vi "Main.vi"() -> ()   [LabVIEW 2012]
doc: "This sample project is built upon the standard state machine template and shows how you could create an application that acquires, analyzes, and presents data. It includes functionality for presenting configuration dialogs, preserving settings between executions, loading and saving data, as well as exporting graph images and text files.\n\nIt is most appropriate for data that is acquired instantly as it does not allow for screen updates mid acquisition nor does it allow for continuous streaming to disk."
uses:
  controls/State.ctl
  controls/Data.ctl
  controls/UI References.ctl
  controls/Graph Data.ctl
  <vilib>/Utility/miscctls.llb/LVAnnotationListTypeDef.ctl
  <vilib>/Utility/miscctls.llb/LVCursorListTypeDef.ctl
  controls/User Specified Data.ctl
  controls/HW Configuration.ctl
  controls/Simulated Signal Type.ctl
  controls/Analysis Configuration.ctl
  controls/New Data Behavior.ctl
  <resource>/Framework/Providers/Wirebird Labs LLC/Deploy/Support/Release Class/Deploy-UpdateService-PromptLevel.ctl
  <resource>/Framework/Providers/Wirebird Labs LLC/Deploy/Support/Update Watcher Class/Deploy-UpdateWatcher.lvclass
  <resource>/Framework/Providers/Wirebird Labs LLC/Deploy/Support/Release Class/Deploy-Release.lvclass
panel:
  in  "Settings":bool
  in  "Snapshot":bool
  in  "Analyze":bool
  in  "Clear":bool
  in  "Stop":bool
  in  "Acquire":bool
  in  "Export":bool
  in  "Save Data":bool
  in  "Load Data":bool
  out "Graph":waveform(dbl)[](graph)
  out "Status Bar":string
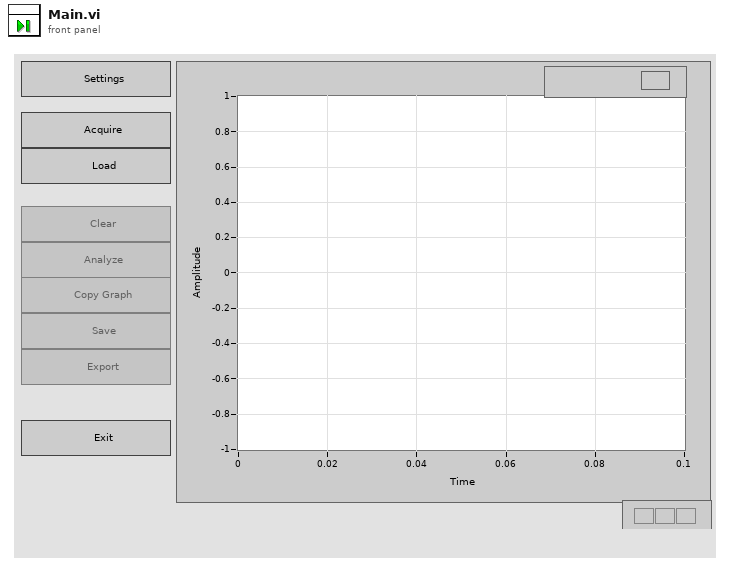
[diagram p1: front panel]
types:
  T1 = typedef "Deploy-Release.lvclass/Deploy-UpdateService-PromptLevel.ctl" = enum16{"Prompt User", "Auto (Show Progress Only)"}
  T2 = typedef "Data.ctl" = cluster{"UI References":T3, "Graph Data":T4, "User Specified":T7}
  T3 = typedef "UI References.ctl" = cluster{"Stop Ref":refnum<vi>, "Save Ref":refnum<vi>, "Open Ref":refnum<vi>, "Export Ref":refnum<vi>, "Acquire Ref":refnum<vi>, "Configure Ref":refnum<vi>, "Graph Ref":refnum<vi>, "Clear Ref":refnum<vi>, "Analyze Ref":refnum<vi>, "Status Ref":refnum<vi>, "Snapshot Ref":refnum<vi>}
  T4 = typedef "Graph Data.ctl" = cluster{"Data":waveform(dbl)[], "Annotation List":T5, "Cursor List":T6, "Analysis Data":waveform(dbl)[]}
  T5 = typedef "LVAnnotationListTypeDef.ctl" = cluster{"Name":string, "Color":u32, "Style":u8, "Point Style":u8, "Name Visible":bool, "Allow Drag":bool, "Annotation Mode":u32, "Plot":i32, "Index":i32, "Position":cluster{"X":dbl, "Y":dbl}, "X Scale":u32, "Y Scale":u32, "Show Arrow":bool, "Lock Name":bool, "Plot Area":i32, "Label Offset":cluster{"X":dbl, "Y":dbl}}[]
  T6 = typedef "LVCursorListTypeDef.ctl" = cluster{"Name":string, "Color":u32, "Style":u8, "Point Style":u8, "Name Visible":bool, "Allow Drag":bool, "Cursor Mode":u32, "Plot":i32, "Index":i32, "Position":cluster{"X":dbl, "Y":dbl}, "X Scale":u32, "Y Scale":u32, "Watch Plots":i32[], "Watch All Plots":bool, "Plot Area":i32, "Label Offset":cluster{"X":dbl, "Y":dbl}}[]
  T7 = typedef "User Specified Data.ctl" = cluster{"Hardware Configuration":T8, "Analysis Configuration":T10, "New Data Behavior":T11}
  T8 = typedef "HW Configuration.ctl" = cluster{"HW Refnum <Replace Me>":string, "Signal Type <Replace Me>":T9}
  T9 = typedef "Simulated Signal Type.ctl" = enum16{"Sine Wave", "Square Wave"}
  T10 = typedef "Analysis Configuration.ctl" = cluster{"Statistics":bool}
  T11 = typedef "New Data Behavior.ctl" = enum16{"Replace", "Overlay", "Append"}
  T12 = typedef "State.ctl" = enum16{"Initialize", "Wait for Event", "Update UI", "Configure", "Acquire", "Load Data", "Save Data", "Clear Data", "Export Data", "Analyze", "Copy Graph", "Stop"}
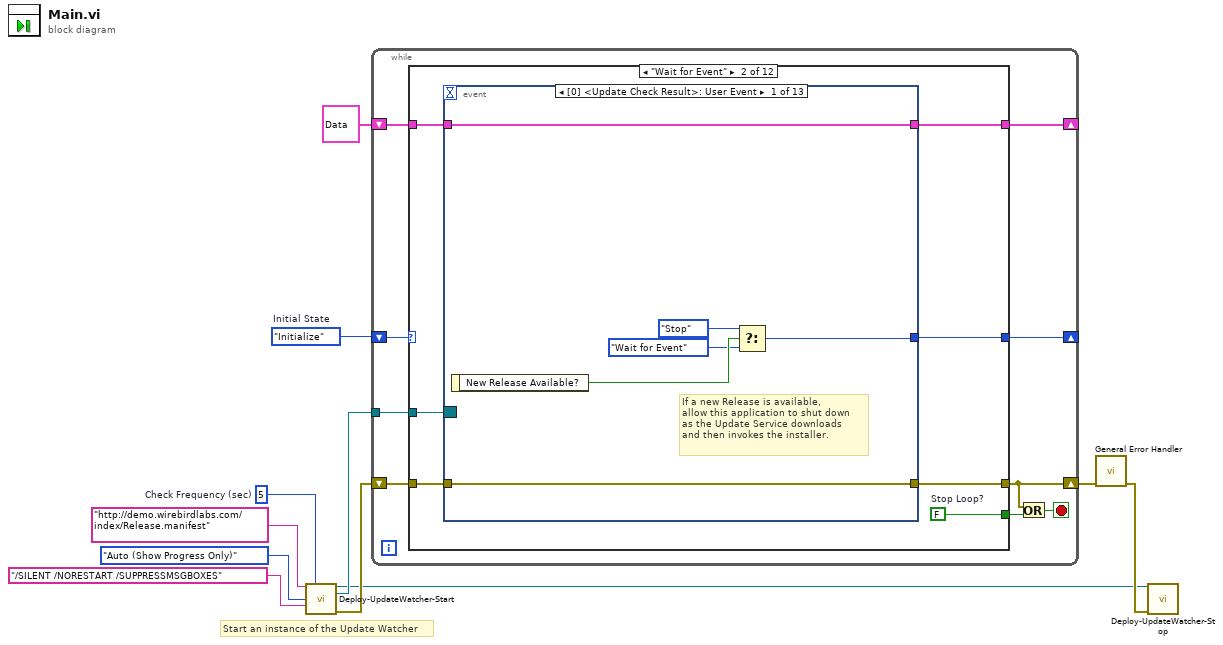
[diagram p0: block diagram]
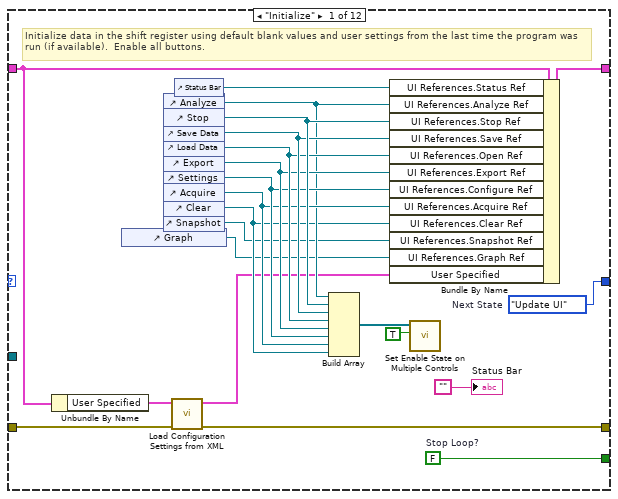
[diagram p2: hidden frame]
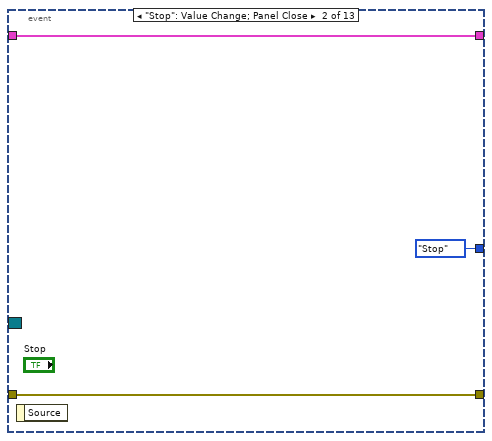
[diagram p3: hidden frame]
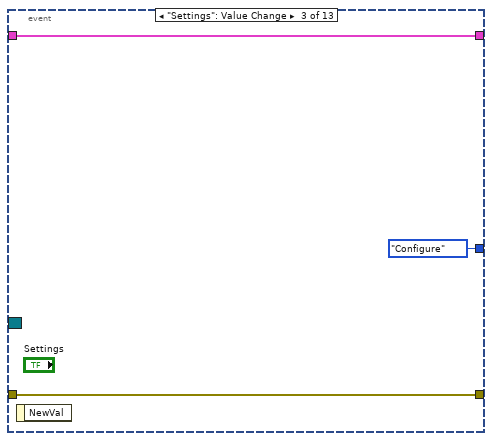
[diagram p4: hidden frame]
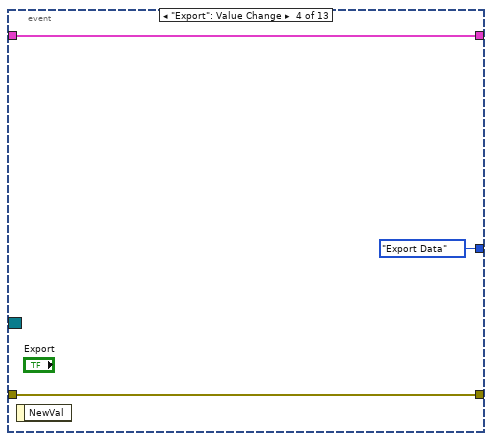
[diagram p5: hidden frame]
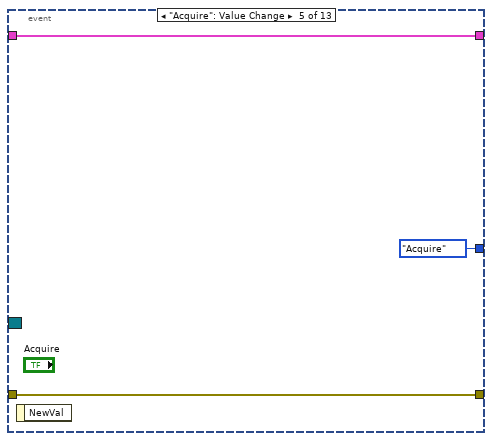
[diagram p6: hidden frame]
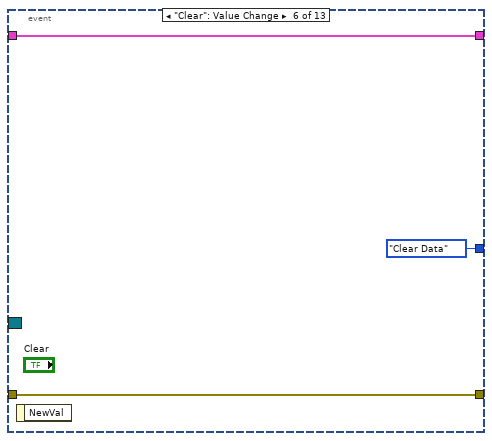
[diagram p7: hidden frame]
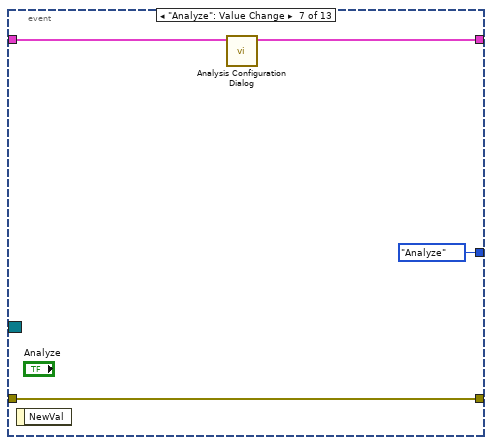
[diagram p8: hidden frame]
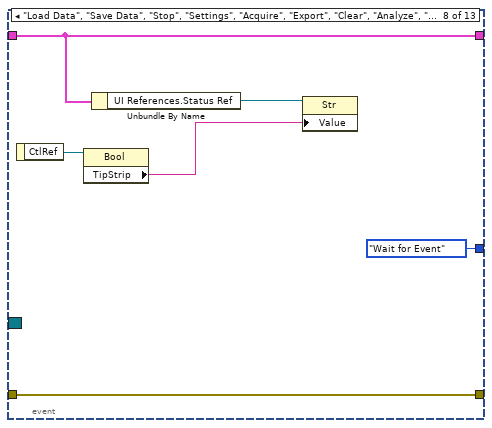
[diagram p9: hidden frame]
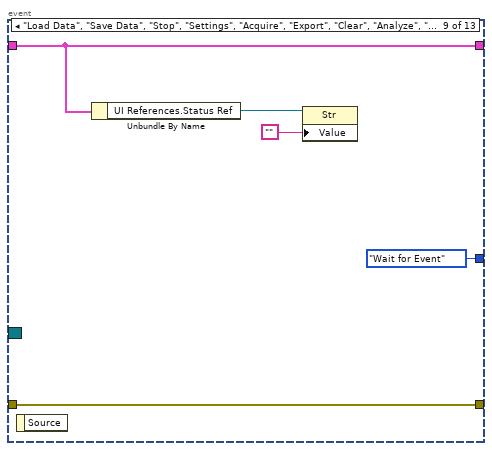
[diagram p10: hidden frame]
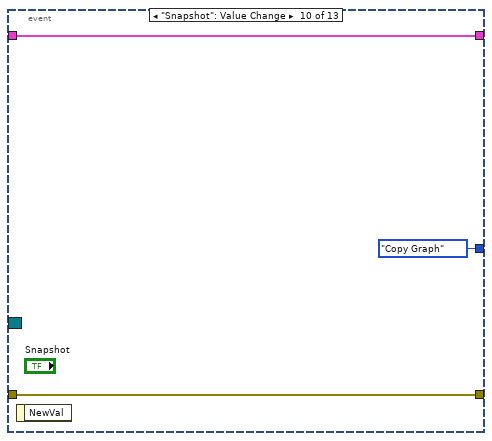
[diagram p11: hidden frame]
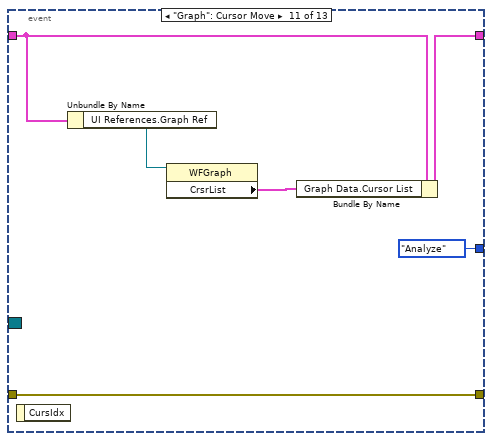
[diagram p12: hidden frame]
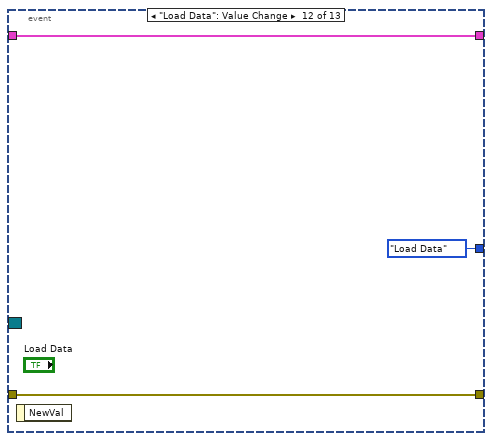
[diagram p13: hidden frame]
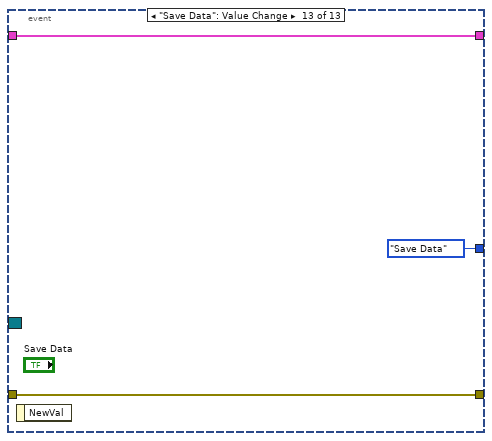
[diagram p14: hidden frame]
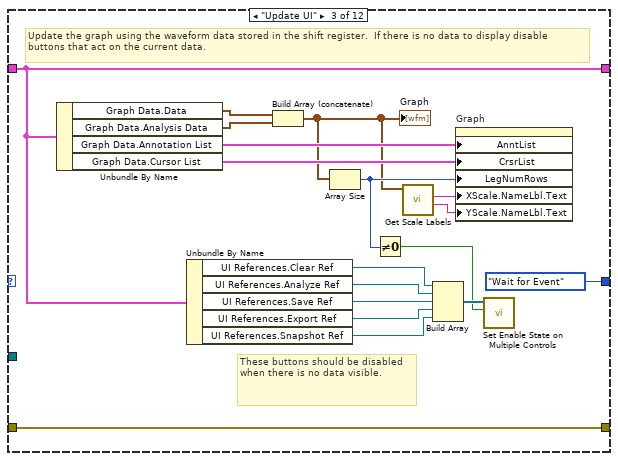
[diagram p15: hidden frame]
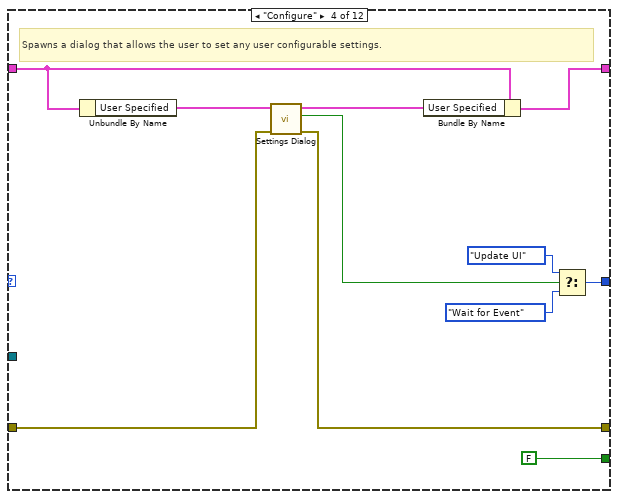
[diagram p16: hidden frame]
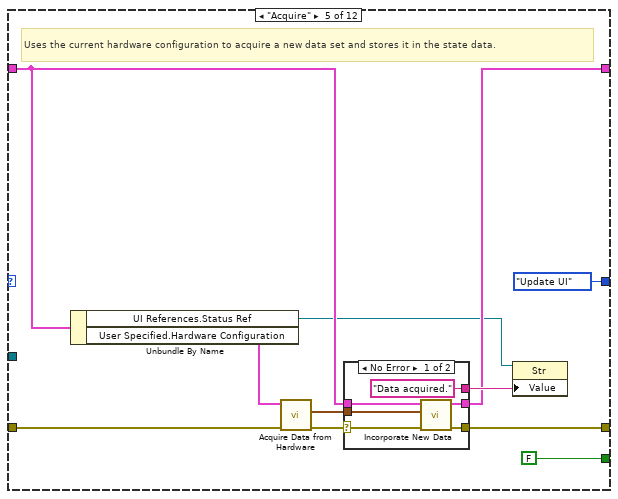
[diagram p17: hidden frame]
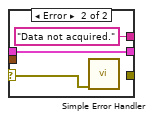
[diagram p18: hidden frame]
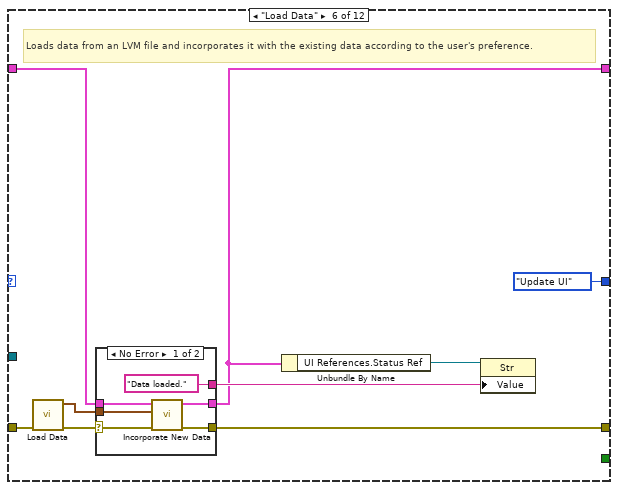
[diagram p19: hidden frame]
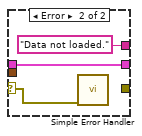
[diagram p20: hidden frame]
diagram:
  w2 = 5  # Check Frequency (sec)
  w11 = State."Initialize"  # Initial State
  # "Start an instance of the Update Watcher"
  n1 = call <resource>:"Deploy-UpdateWatcher-Start.vi"("Manifest URI"="http://demo.wirebirdlabs.com/index/Release.manifest", "Check Frequency (sec)"=w2, "Prompt Level"=Deploy-UpdateService-PromptLevel."Auto (Show Progress Only)", "Installer Command Line Parameters"="/SILENT /NORESTART /SUPPRESSMSGBOXES") -> (4:"Update Watcher"=w3:refnum<class "Deploy-UpdateWatcher.lvclass">, 6:"Update Watcher"=w8:refnum<event-registration>, "error out"=w6:errorcluster)  [unwired: 9 in]
  n2 = while {
    shift-right: [w19] -> _
    shift-left: w11 -> [w20]
    shift-right: [w17] -> _
    shift-left: T2 {"UI References"={"Stop Ref"=refnum, "Save Ref"=refnum, "Open Ref"=refnum, "Export Ref"=refnum, "Acquire Ref"=refnum, "Configure Ref"=refnum, "Graph Ref"=refnum, "Clear Ref"=refnum, "Analyze Ref"=refnum, "Status Ref"=refnum, "Snapshot Ref"=refnum}, "Graph Data"={"Data"=[], "Annotation List"=[], "Cursor List"=[], "Analysis Data"=[]}, "User Specified"={"Hardware Configuration"={"HW Refnum <Replace Me>"="", "Signal Type <Replace Me>"=enum."Sine Wave"}, "Analysis Configuration"={"Statistics"=FALSE}, "New Data Behavior"=enum."Replace"}} ("Data") -> [w18]
    shift-right: [w13] -> w9
    shift-left: w6 -> [w16]
    tunnel: w8 -> [w12]
    stop <- w14 stop-if-true
    n3 = case shown="\"Wait for Event\"" w20 {
      tunnel: [w42 w49 State."Wait for Event" ("(Value Not Used)") w122 State."Update UI" ("Next State") State."Update UI" ("(Value Not Used)") State."Wait for Event" ("(Value Not Used)") State."Wait for Event" ("(Value Not Used)") State."Update UI" ("(Value Not Used)") State."Update UI" ("(Value Not Used)") State."Wait for Event" ("(Value Not Used)") w212] -> w19
      tunnel: [w41 w48 _ FALSE ("Stop Loop?") FALSE ("Stop Loop?") _ _ _ _ _ _ w211] -> w15
      tunnel: w18 -> [w32 w47 w115 w128 w135 w158 w171 w183 w194 w197 w203 w209]
      tunnel: [w40 w46 w115 w127 w134 w152 w171 w183 w193 w197 w203 w209] -> w17
      tunnel: w16 -> [w30 w45 w118 w126 w137 w157 w173 w186 w196 w198 w202 w206]
      tunnel: [w29 w44 w118 w125 w130 w156 w169 w180 w196 w198 w201 w205] -> w13
      tunnel: w12 -> [_ w43 _ _ _ _ _ _ _ _ _ _]
      frame "Initialize" {
        w41 = FALSE  # Stop Loop?
        w42 = State."Update UI"  # Next State
        # "Initialize data in the shift register using default blank values and user settings from the last time the program was run (if available).  Enable all buttons."
        n4 = Unbundle By Name(w32) -> ("User Specified"=w31:T7)
        n5 = control-ref of="Graph"() -> (w21:refnum<vi>)
        n6 = control-ref of="Analyze"() -> (w28:refnum<vi>)
        n7 = control-ref of="Stop"() -> (w39:refnum<vi>)
        n8 = control-ref of="Save Data"() -> (w38:refnum<vi>)
        n9 = control-ref of="Load Data"() -> (w37:refnum<vi>)
        n10 = control-ref of="Export"() -> (w36:refnum<vi>)
        n11 = control-ref of="Settings"() -> (w35:refnum<vi>)
        n12 = control-ref of="Acquire"() -> (w34:refnum<vi>)
        n13 = control-ref of="Clear"() -> (w26:refnum<vi>)
        n14 = control-ref of="Snapshot"() -> (w22:refnum<vi>)
        n15 = call "Load Configuration Settings from XML.vi"("error in (no error)"=w30, "User Configuration in"=w31) -> ("error out"=w29:errorcluster, "User Configuration out"=w24:T7)  [unwired: 8 in]
        n16 = control-ref of="Status Bar"() -> (w27:refnum<vi>)
        n17 = Build Array(w28, w39, w38, w37, w36, w35, w34, w26) -> (w33:refnum<vi>[])
        n18 = Bundle By Name(cluster=w32, "UI References.Status Ref"=w27, "UI References.Analyze Ref"=w28, "UI References.Stop Ref"=w39, "UI References.Save Ref"=w38, "UI References.Open Ref"=w37, "UI References.Export Ref"=w36, "UI References.Configure Ref"=w35, "UI References.Acquire Ref"=w34, "UI References.Clear Ref"=w26, "UI References.Snapshot Ref"=w22, "UI References.Graph Ref"=w21, "User Specified"=w24) -> (w40:T2)
        n19 = call "Set Enable State on Multiple Controls.vi"("Enable?"=TRUE, "Controls"=w33) -> ()  [unwired: 10 in]
        "Status Bar" <- "" ("Status Bar")
      }
      frame "Wait for Event" {
        w48 = FALSE  # Stop Loop?
        n20 = event shown="[0] <Update Check Result>: User Event" {
          selector: w43 -> [_ _ _ _ _ _ _ _ _ _ _ _ _]
          dyn-events: _ -> [_ _ _ _ _ _ _ _ _ _ _ _ _]
          timeout: _ -> [_ _ _ _ _ _ _ _ _ _ _ _ _]
          tunnel: [w51 State."Stop" ("Next State") State."Configure" ("Next State") State."Export Data" ("Next State") State."Acquire" ("Next State") State."Clear Data" ("Next State") State."Analyze" ("Next State") State."Wait for Event" ("Next State") State."Wait for Event" ("Next State") State."Copy Graph" ("Next State") State."Analyze" ("Next State") State."Load Data" ("Next State") State."Save Data" ("Next State")] -> w49
          tunnel: w47 -> [w55 w57 w61 w64 w67 w70 w72 w78 w84 w88 w89 w96 w99]
          tunnel: [w55 w57 w61 w64 w67 w70 w71 w78 w84 w88 w92 w96 w99] -> w46
          tunnel: w45 -> [w54 w56 w60 w63 w66 w69 w74 w80 w85 w87 w94 w95 w98]
          tunnel: [w54 w56 w60 w63 w66 w69 w74 w80 w85 w87 w94 w95 w98] -> w44
          event User Event {
            # "If a new Release is available,\nallow this application to shut down\nas the Update Service downloads\nand then invokes the installer."
            n21 = event-data() -> ("New Release Available?"=w53:bool)  [unwired: 1 in]
            n22 = Select(t=State."Stop" ("Next State"), s=w53, f=State."Wait for Event") -> (s? t:f=w51:T12)
          }
          event "Stop": Value Change; Panel Close {
            n23 = event-data() -> ()  [unwired: 1 in, 1 out]
          }
          event "Settings": Value Change {
            n24 = event-data() -> ()  [unwired: 1 in, 1 out]
          }
          event "Export": Value Change {
            n25 = event-data() -> ()  [unwired: 1 in, 1 out]
          }
          event "Acquire": Value Change {
            n26 = event-data() -> ()  [unwired: 1 in, 1 out]
          }
          event "Clear": Value Change {
            n27 = event-data() -> ()  [unwired: 1 in, 1 out]
          }
          event "Analyze": Value Change {
            n28 = event-data() -> ()  [unwired: 1 in, 1 out]
            n29 = call "Analysis Configuration Dialog.vi"("Data in"=w72) -> ("Data out"=w71:T2)  [unwired: 10 in]
          }
          event "Load Data", "Save Data", "Stop", "Settings", "Acquire", "Export", "Clear", "Analyze", "Snapshot": Mouse Enter {
            n30 = event-data() -> ("CtlRef"=w79:refnum<vi>)  [unwired: 1 in]
            n31 = property class="Bool"(reference=w79) -> ("TipStrip"=w76:string)  [unwired: 1 in, 2 out]
            n32 = Unbundle By Name(w78) -> ("UI References.Status Ref"=w77:refnum<vi>)
            n33 = property class="Str"(reference=w77, "Value"=w76) -> ()  [unwired: 1 in, 2 out]
          }
          event "Load Data", "Save Data", "Stop", "Settings", "Acquire", "Export", "Clear", "Analyze", "Snapshot": Mouse Leave {
            n34 = event-data() -> ()  [unwired: 1 in, 1 out]
            n35 = Unbundle By Name(w84) -> ("UI References.Status Ref"=w83:refnum<vi>)
            n36 = property class="Str"(reference=w83, "Value"="") -> ()  [unwired: 1 in, 2 out]
          }
          event "Snapshot": Value Change {
            n37 = event-data() -> ()  [unwired: 1 in, 1 out]
          }
          event "Graph": Cursor Move {
            n38 = event-data() -> ()  [unwired: 1 in, 1 out]
            n39 = Unbundle By Name(w89) -> ("UI References.Graph Ref"=w91:refnum<vi>)
            n40 = property class="WFGraph"(reference=w91) -> ("CrsrList"=w90:T6)  [unwired: 1 in, 2 out]
            n41 = Bundle By Name(cluster=w89, "Graph Data.Cursor List"=w90) -> (w92:T2)
          }
          event "Load Data": Value Change {
            n42 = event-data() -> ()  [unwired: 1 in, 1 out]
          }
          event "Save Data": Value Change {
            n43 = event-data() -> ()  [unwired: 1 in, 1 out]
          }
        }
      }
      frame "Update UI" {
        # "These buttons should be disabled when there is no data visible."
        # "Update the graph using the waveform data stored in the shift register.  If there is no data to display disable buttons that act on the current data."
        n44 = Unbundle By Name(w115) -> ("Graph Data.Data"=w111:waveform(dbl)[], "Graph Data.Analysis Data"=w101:waveform(dbl)[], "Graph Data.Annotation List"=w116:T5, "Graph Data.Cursor List"=w112:T6)
        n45 = Unbundle By Name(w115) -> ("UI References.Clear Ref"=w107:refnum<vi>, "UI References.Analyze Ref"=w106:refnum<vi>, "UI References.Save Ref"=w114:refnum<vi>, "UI References.Export Ref"=w104:refnum<vi>, "UI References.Snapshot Ref"=w105:refnum<vi>)
        n46 = Build Array (concatenate)(w111, w101) -> (w109:waveform(dbl)[])
        "Graph" <- w109
        n47 = Array Size(array=w109) -> (size(s)=w110:i32)
        n48 = Not Equal To 0?(x=w110) -> (x != 0?=w108:bool)
        n49 = call "Get Scale Labels.vi"("Array of Waveforms"=w109) -> ("Y Scale Label Text"=w102:string, "X Scale Label Text"=w103:string)  [unwired: 9 in]
        n50 = Build Array(w107, w106, w114, w104, w105) -> (w113:refnum<vi>[])
        n51 = property on="Graph" class="WFGraph (strict)"("AnntList"=w116, "CrsrList"=w112, "LegNumRows"=w110, "XScale.NameLbl.Text"=w103, "YScale.NameLbl.Text"=w102) -> ()  [unwired: 2 in, 2 out]
        n52 = call "Set Enable State on Multiple Controls.vi"("Enable?"=w108, "Controls"=w113) -> ()  [unwired: 10 in]
      }
      frame "Configure" {
        # "Spawns a dialog that allows the user to set any user configurable settings."
        n53 = Unbundle By Name(w128) -> ("User Specified"=w120:T7)
        n54 = call "Settings Dialog.vi"("error in (no error)"=w126, "Configuration in"=w120) -> ("error out"=w125:errorcluster, "UI Refresh Needed?"=w124:bool, "Configuration out"=w119:T7)  [unwired: 7 in]
        n55 = Bundle By Name(cluster=w128, "User Specified"=w119) -> (w127:T2)
        n56 = Select(t=State."Update UI" ("Next State if true"), s=w124, f=State."Wait for Event" ("Next State if false")) -> (s? t:f=w122:T12)
      }
      frame "Acquire" {
        # "Uses the current hardware configuration to acquire a new data set and stores it in the state data."
        n57 = Unbundle By Name(w135) -> ("UI References.Status Ref"=w131:refnum<vi>, "User Specified.Hardware Configuration"=w138:T8)
        n58 = call "Acquire Data from Hardware.vi"("error in (no error)"=w137, "Hardware Configuration"=w138) -> ("error out"=w132:errorcluster, "Graph Data"=w133:waveform(dbl)[])  [unwired: 7 in]
        n59 = case shown="No Error" w132 {
          selector: w132 -> [w143 w148]
          tunnel: w135 -> [w142 w149]
          tunnel: [w146 w149] -> w134
          tunnel: [w145 _] -> w130
          tunnel: w133 -> [w144 _]
          tunnel: ["Data acquired." ("Data acquired") "Data not acquired." ("Data not acquired")] -> w136
          frame No Error {
            n60 = call "Incorporate New Data.vi"("error in (no error)"=w143, "New Graph Data"=w144, "Data in"=w142) -> ("error out"=w145:errorcluster, "Data out"=w146:T2)  [unwired: 7 in]
          }
          frame Error {
            n61 = call <vilib>:"Simple Error Handler.vi"("error in (no error)"=w148) -> ()  [unwired: 4 in, 5 out]
          }
        }
        n62 = property class="Str"(reference=w131, "Value"=w136) -> ()  [unwired: 1 in, 2 out]
      }
      frame "Load Data" {
        # "Loads data from an LVM file and incorporates it with the existing data according to the user's preference."
        n63 = call "Load Data.vi"("error in (no error)"=w157) -> ("error out"=w154:errorcluster, "New Graph Data"=w151:waveform(dbl)[])  [unwired: 9 in]
        n64 = case shown="No Error" w154 {
          selector: w154 -> [w161 w166]
          tunnel: w158 -> [w160 w167]
          tunnel: [w164 w167] -> w152
          tunnel: [w163 _] -> w156
          tunnel: w151 -> [w162 _]
          tunnel: ["Data loaded." ("Data loaded") "Data not loaded." ("Data not loaded")] -> w153
          frame No Error {
            n65 = call "Incorporate New Data.vi"("error in (no error)"=w161, "New Graph Data"=w162, "Data in"=w160) -> ("error out"=w163:errorcluster, "Data out"=w164:T2)  [unwired: 7 in]
          }
          frame Error {
            n66 = call <vilib>:"Simple Error Handler.vi"("error in (no error)"=w166) -> ()  [unwired: 4 in, 5 out]
          }
        }
        n67 = Unbundle By Name(w152) -> ("UI References.Status Ref"=w150:refnum<vi>)
        n68 = property class="Str"(reference=w150, "Value"=w153) -> ()  [unwired: 1 in, 2 out]
      }
      frame "Save Data" {
        # "Saves the existing measurement data to an LVM file."
        n69 = Unbundle By Name(w171) -> ("UI References.Status Ref"=w170:refnum<vi>, "Graph Data.Data"=w174:waveform(dbl)[])
        n70 = call "Save Data.vi"("error in (no error)"=w173, "Data"=w174) -> ("error out"=w172:errorcluster)  [unwired: 9 in]
        n71 = case shown="No Error" w172 {
          selector: w172 -> [w176 w179]
          tunnel: ["Data saved." ("Data saved") "Data not saved." ("Data not saved")] -> w168
          tunnel: [w176 _] -> w169
          frame No Error {
          }
          frame Error {
            n72 = call <vilib>:"Simple Error Handler.vi"("error in (no error)"=w179) -> ()  [unwired: 4 in, 5 out]
          }
        }
        n73 = property class="Str"(reference=w170, "Value"=w168) -> ()  [unwired: 1 in, 2 out]
      }
      frame "Export Data" {
        # "Exports the currently loaded measurement and analysis data to a text file that can be imported into a spreadsheet or other application."
        n74 = Unbundle By Name(w183) -> ("UI References.Status Ref"=w181:refnum<vi>, "Graph Data"=w182:T4)
        n75 = call "Export Data.vi"("error in (no error)"=w186, "Graph Data"=w182) -> ("error out"=w184:errorcluster)  [unwired: 9 in]
        n76 = case shown="No Error" w184 {
          selector: w184 -> [w188 w191]
          tunnel: ["Data exported." ("Data exported") "Data not exported." ("Data not exported")] -> w185
          tunnel: [w188 _] -> w180
          frame No Error {
          }
          frame Error {
            n77 = call <vilib>:"Simple Error Handler.vi"("error in (no error)"=w191) -> ()  [unwired: 4 in, 5 out]
          }
        }
        n78 = property class="Str"(reference=w181, "Value"=w185) -> ()  [unwired: 1 in, 2 out]
      }
      frame "Clear Data" {
        # "Clears the data currently in the graph."
        n79 = Bundle By Name(cluster=w194, "Graph Data"=T4 {"Data"=[], "Annotation List"=[], "Cursor List"=[], "Analysis Data"=[]} ("Graph")) -> (w193:T2)
      }
      frame "Analyze" {
        # "Code Recommended - Add your own signal analysis here."
        # "Analyzes the measurement data."
        n80 = Unbundle By Name(w197) -> ("Graph Data"=w199:T4)
        n81 = call "Statistical Analysis.vi"("Graph Data In"=w199) -> ()  [unwired: 8 in, 2 out]
      }
      frame "Copy Graph" {
        # "Places an image of the graph on the clipboard for pasting into reports or emails."
        n82 = call "Copy Graph to Clipboard.vi"("error in (no error)"=w202, "Graph Data"=w203) -> ("error out"=w201:errorcluster)  [unwired: 9 in]
      }
      frame "Stop" {
        w211 = TRUE  # Stop Loop?
        w212 = State."Stop"  # (Value Not Used)
        # "Saves the users settings to an XML file and stops execution."
        # "The state value is not used here since this is the last iteration of the state machine loop"
        n83 = Unbundle By Name(w209) -> ("UI References.Status Ref"=w207:refnum<vi>, "User Specified"=w210:T7)
        n84 = call "Save Configuration Settings to XML.vi"("error in (no error)"=w206, "User Configuration"=w210) -> ("error out"=w205:errorcluster)  [unwired: 9 in]
        n85 = property class="Str"(reference=w207, "Value"="Stopped." ("Stopped")) -> ()  [unwired: 1 in, 2 out]
      }
    }
    n86 = Or(x=w13, y=w15) -> (x .or. y?=w14:bool)
  }
  n87 = call <vilib>:"General Error Handler.vi"("error in (no error)"=w9) -> ("error out"=w7:errorcluster)  [unwired: 10 in, 4 out]
  n88 = call <resource>:"Deploy-UpdateWatcher-Stop.vi"("Update Watcher"=w3, "error in"=w7) -> ()  [unwired: 13 in, 1 out]
